vi "L Command.vi"(8 "error in (no error)":errorcluster, 11 "PSP-405 resource in":refnum<visa-resource-name>) -> (0 "error out":errorcluster, 2 "response":T1, 3 "PSP-405 resource out":refnum<visa-resource-name>, 4 "raw response":string)   [LabVIEW 2017, in "GW Instek PSP-405.lvlib"]
doc: "The L query returns all the status values of the power supply."
uses:
  GW Instek PSP-405.lvlib
  CTLs/L Command Response.ctl
  CTLs/Values.ctl
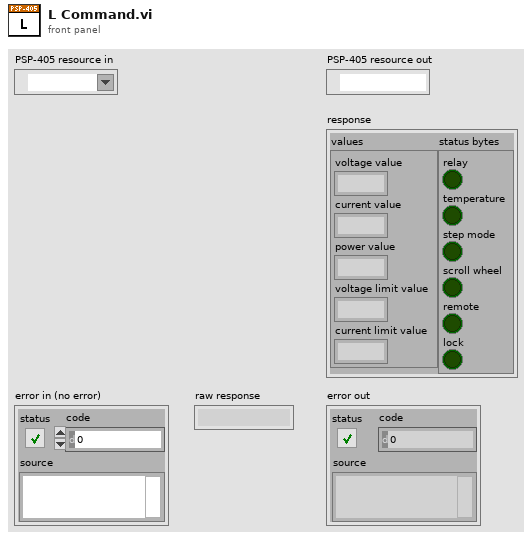
[diagram p1: front panel]
types:
  T1 = typedef "GW Instek PSP-405.lvlib/L Command Response.ctl" = cluster{"values":T2, "status bytes":cluster{"relay":bool, "temperature":bool, "step mode":bool, "scroll wheel":bool, "remote":bool, "lock":bool}}
  T2 = typedef "GW Instek PSP-405.lvlib/Values.ctl" = cluster{"voltage value":dbl, "current value":dbl, "power value":dbl, "voltage limit value":dbl, "current limit value":dbl}
  T3 = cluster{"f1":bool, "f2":bool, "f3":bool, "f4":bool, "f5":bool, "f6":bool}
  T4 = cluster{"[0]":dbl, "[1]":dbl, "[2]":dbl, "[3]":dbl, "[4]":dbl}
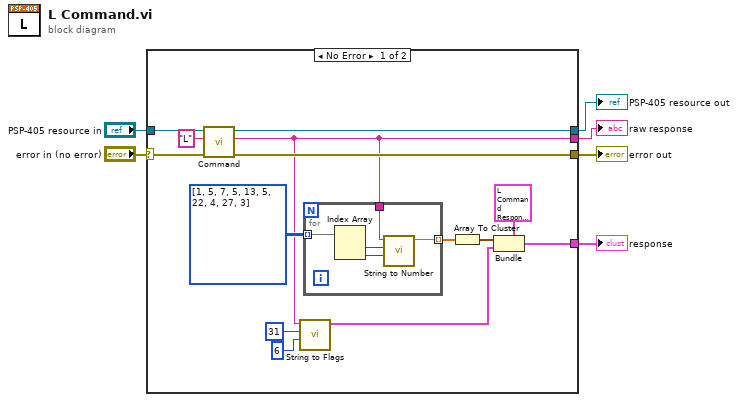
[diagram p0: block diagram]
diagram:
  n1 = case shown="No Error" "error in (no error)" {
    selector: "error in (no error)" -> [w14 w27]
    tunnel: "PSP-405 resource in" -> [w19 w26]
    tunnel: [w10 _] -> w5
    tunnel: [w16 _] -> w4
    tunnel: [w20 w27] -> w3
    tunnel: [w13 w26] -> w1
    frame No Error {
      n2 = call "Command.vi"("error in (no error)"=w14, "cmd"="L", "PSP-405 resource in"=w19) -> ("error out"=w20:errorcluster, "response"=w10:string, "PSP-405 resource out"=w13:refnum<visa-resource-name>)  [unwired: 6 in]
      n3 = call "String to Flags.vi"("length"=6 ("length (rest)"), "offset"=31 ("offset (0)"), "string"=w10) -> ("flags"=w8:T3)  [unwired: 8 in]
      n4 = for {
        tunnel: i32[][] [[1, 5], [7, 5], [13, 5], [22, 4], [27, 3]] -> [w25] mode=indexing
        tunnel: [w22] -> w9 mode=indexing
        tunnel: w10 -> [w21]
        n5 = Index Array(array=w25) -> (element #1=w24:i32, element #2=w23:i32)  [unwired: 2 in]
        n6 = call "String to Number.vi"("length"=w23, "offset"=w24, "string"=w21) -> ("numeric"=w22:dbl)  [unwired: 8 in]
      }
      n7 = Array To Cluster(array=w9) -> (cluster=w7:T4)
      n8 = Bundle(cluster=T1 {"values"={"voltage value"=0.0, "current value"=0.0, "power value"=0.0, "voltage limit value"=0.0, "current limit value"=0.0}, "status bytes"={"relay"=FALSE, "temperature"=FALSE, "step mode"=FALSE, "scroll wheel"=FALSE, "remote"=FALSE, "lock"=FALSE}} ("response"), "values"=w7, "status bytes"=w8) -> (w16:T1)
    }
    frame Error {
    }
  }
  "error out" <- w3
  "raw response" <- w5
  "response" <- w4
  "PSP-405 resource out" <- w1
